vi "camera FGV.vi"(4 "Operation":enum16{"Init", "Get", "Set"}(ring)=enum."Get", 8 "error in":errorcluster, 11 "camera in":u32) -> (0 "error out":errorcluster, 2 "camera out":u32)   [LabVIEW 2021]
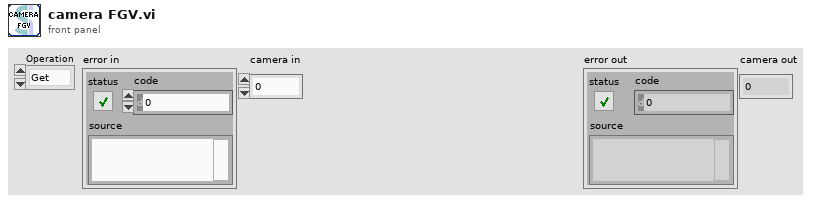
[diagram p1: front panel]
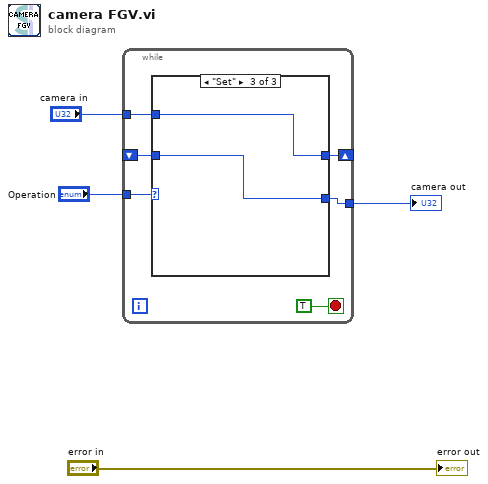
[diagram p0: block diagram]
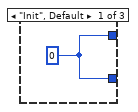
[diagram p2: hidden frame]
diagram:
  n1 = while {
    tunnel: "Operation" -> [w9]
    shift-right: [w8] -> _
    shift-left: _ -> [w7]
    tunnel: [w6] -> w2
    tunnel: "camera in" -> [w5]
    stop <- TRUE stop-if-true
    n2 = case shown="\"Set\"" w9 {
      tunnel: [w11 w12 w14] -> w8
      tunnel: w7 -> [_ w12 w13]
      tunnel: [w11 w12 w13] -> w6
      tunnel: w5 -> [_ _ w14]
      frame "Init", Default {
        w11 = u32 0
      }
      frame "Get" {
      }
      frame "Set" {
      }
    }
  }
  "camera out" <- w2
  "error out" <- "error in"
